vi "FPGA Main.vi"() -> ()   [LabVIEW 2018]
uses:
  <vilib>/Platform/TimedLoop/XDataNode/timing_clust.ctl
  <vilib>/Platform/TimedLoop/XDataNode/nitl_modes.ctl
  <vilib>/Platform/TimedLoop/XDataNode/wakeup.ctl
  <vilib>/rvi/Emulation/niFpgaGetClockAttributes.vi
  <vilib>/rvi/Emulation/niFpgaSctlEmulationGetInTimedLoop.vi
  <vilib>/rvi/Emulation/niFpgaEmulationReportErrorSimple.vi
  <vilib>/rvi/eio/common/nirviEmuTemplateMethod_errors.vi
  <vilib>/rvi/Emulation/niFpgaCriticalErrorInLSC.vi
  <vilib>/rvi/Emulation/niFpgaProcessEmulError.vi
  <vilib>/Platform/TimedLoop/XDataNode/XDataNode.xnode
  <vilib>/eio/EIONode/EIONode.xnode
  <vilib>/Platform/TimedLoop/XDataNode/XDNodeRunTimeDep.lvlib
panel:
  in  "Sample rate (Ticks) 1":i64=80
  in  "Sample rate (Ticks) 2":i64=80
  in  "Lower Threshold 2":i64
  in  "Anlalog input 2":refnum<k21>="ConnectorA/AI2"
  in  "Lower Threshold 1":i64
  in  "Anlalog input 1":refnum<k21>="ConnectorA/AI1"
  in  "chieu 2":bool=TRUE
  in  "chieu 1":bool=TRUE
  in  "start 2":bool
  in  "Fan Rotation 2":i64
  in  "Asix Rotation":i64
  in  "start 1":bool
  in  "reset count":bool
  out "coincedience":bool
  in  "reset":bool=TRUE
  in  "Gated-2  (ns)2":i64
  in  "Delay-1 (ns)":i64
  out "Count":i64
  out "signal out 2":bool
  out "signal out":bool
  in  "Delay-2 (ns)":i64
  in  "Gated-1  (ns)":i64
  in  "Digital input 2":refnum<k21>="ConnectorA/DIO1"
  in  "Digital input 1":refnum<k21>="ConnectorA/DIO0"
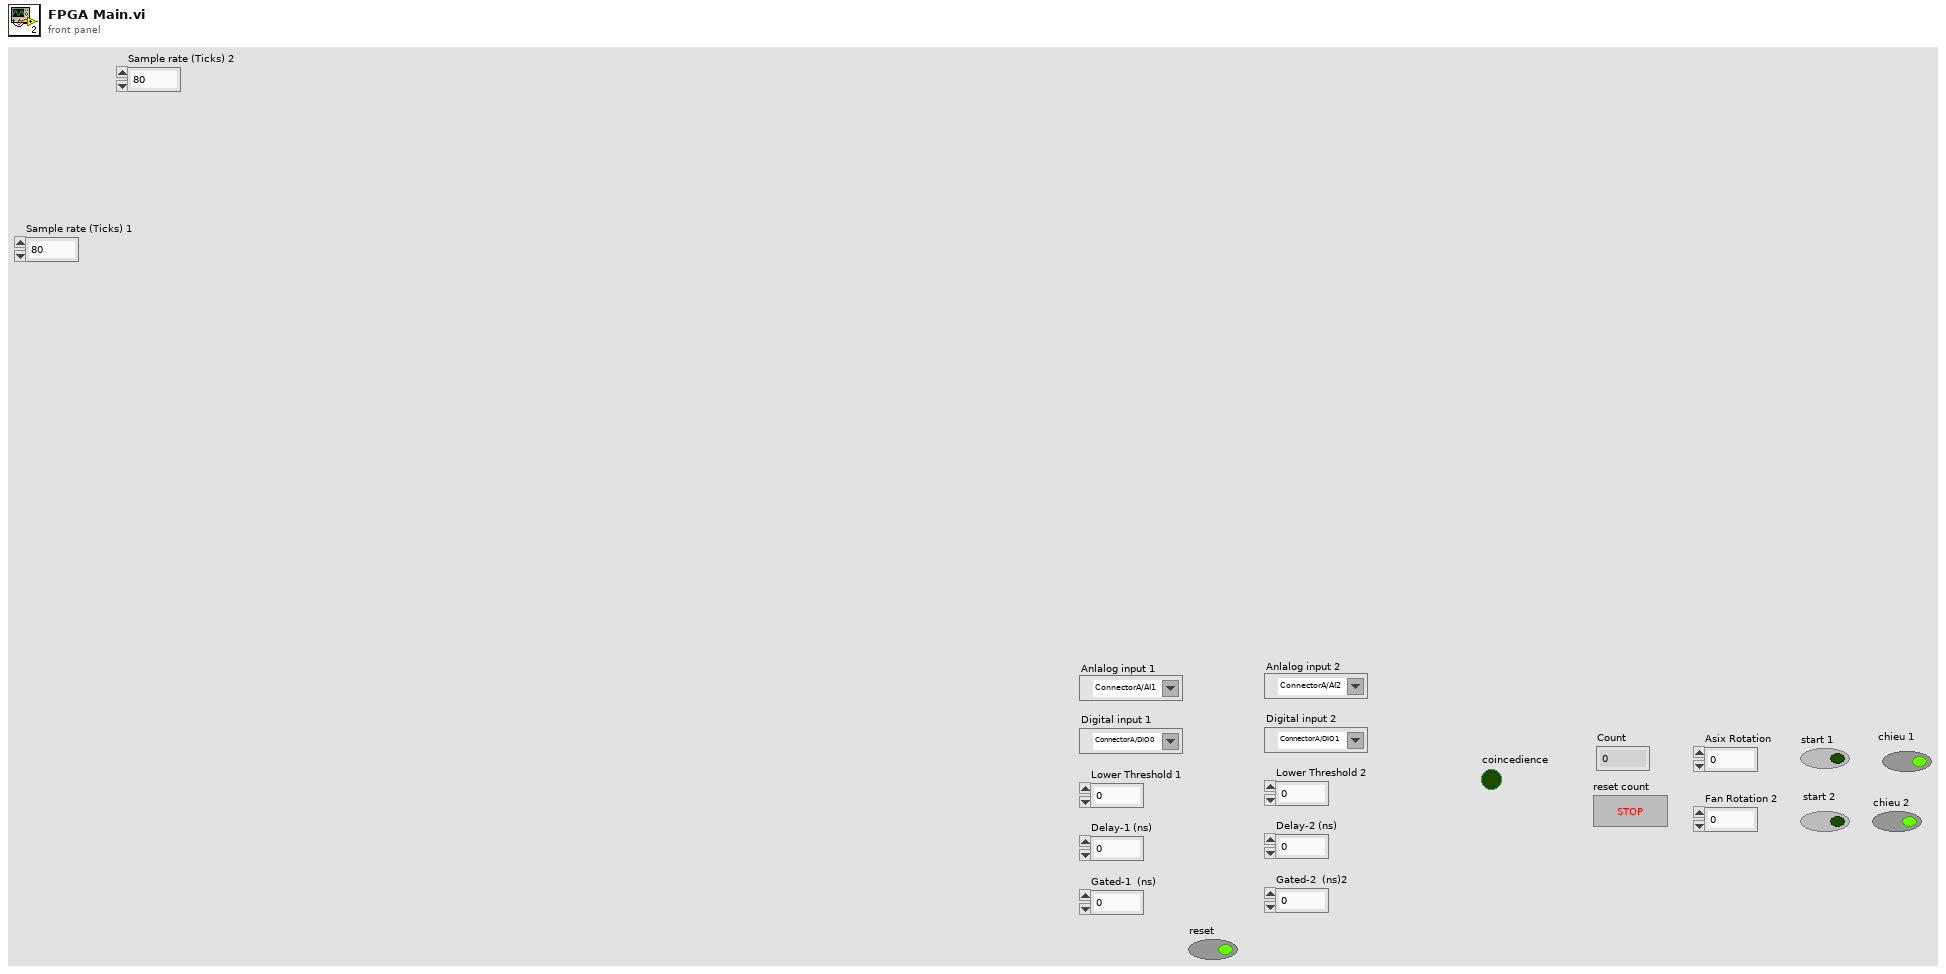
[diagram p1: front panel]
types:
  T1 = typedef "XDNodeRunTimeDep.lvlib/timing_clust.ctl" = cluster{"Expected End [f-1]":u64, "Actual End [f-1]":u64, "Finished Late? [f-1]":bool, "Expected End [i-1]":u64, "Actual End [i-1]":u64, "Finished Late? [i-1]":bool, "Expected Start [i]":u64, "Actual Start [i]":u64, "Expected Start [f]":u64, "Actual Start [f]":u64, "Source Name":string, "Structure Name":string, "Period":i64, "Deadline":i64, "Offset":i64, "Start":i64, "Priority":i32, "Timeout":i32, "Mode":T2, "Wakeup Reason":T3, "Error":errorcluster, "Source Type":string, "Secondary Source Type":string, "Global End Time":u64, "Global Start Time":u64, "Frame Duration":u64, "Iteration Duration":u64, "Assigned CPU":i32, "I/O Scan Engine Mode":u32}
  T2 = typedef "XDNodeRunTimeDep.lvlib/nitl_modes.ctl" = enum32{"No Change", "Process missed periods, maintain original phase", "Discard missed periods, maintain original phase", "Process missed periods, ignore original phase", "Discard missed periods, ignore original phase"}
  T3 = typedef "XDNodeRunTimeDep.lvlib/wakeup.ctl" = enum32{"Normal", "Aborted", "Asynchronous wakeup", "Timing source error", "Timed loop error", "Timeout"}
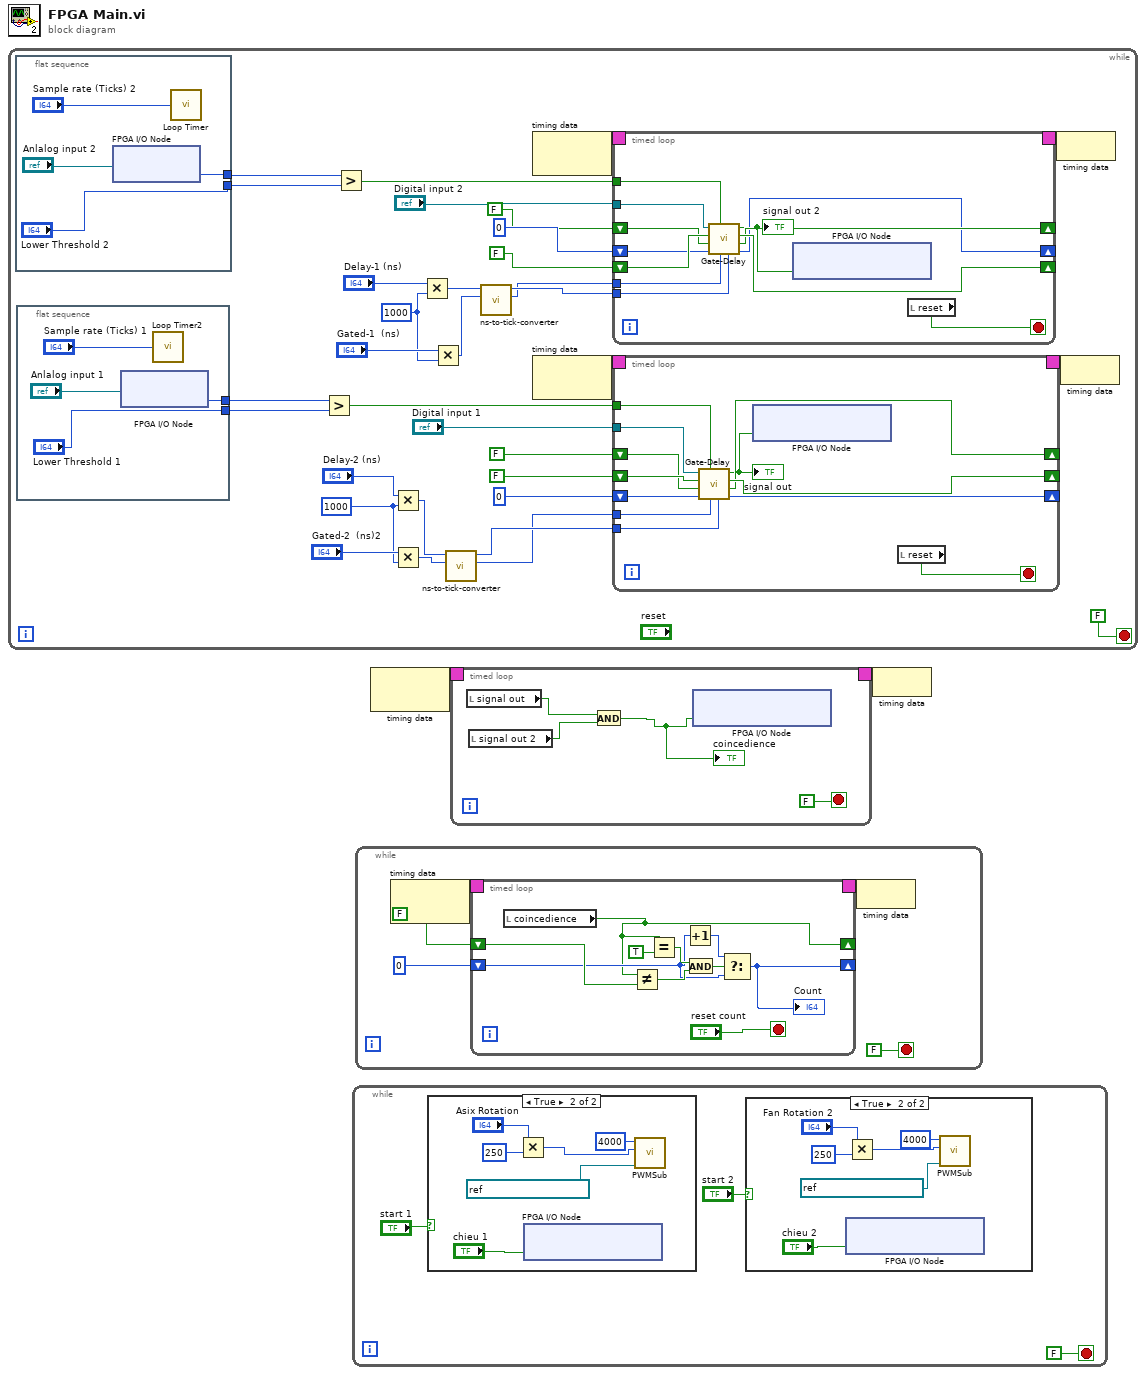
[diagram p0: block diagram]
diagram:
  n1 = while {
    stop <- FALSE stop-if-true
    w10 = i64 1000 ("y")
    w13 = i64 1000 ("y")
    n2 = flat-sequence {
      tunnel: [w40] -> w3
      tunnel: ["Lower Threshold 2"] -> w5
      frame #0 {
        n3 = xnode "FPGA I/O Node"("FPGA I/O In"="Anlalog input 2") -> ("I/O Item"=w40:u16)  [unwired: 1 out]
        n4 = call "Loop Timer"("Count(Ticks)"="Sample rate (Ticks) 2") -> ()  [unwired: 1 out]
      }
    }
    n5 = flat-sequence {
      tunnel: ["Lower Threshold 1"] -> w8
      tunnel: [w37] -> w7
      frame #0 {
        n6 = xnode "FPGA I/O Node"("FPGA I/O In"="Anlalog input 1") -> ("I/O Item"=w37:u16)  [unwired: 1 out]
        n7 = call "Loop Timer2"("Count(Ticks)"="Sample rate (Ticks) 1") -> ()  [unwired: 1 out]
      }
    }
    n8 = Greater?(x=w7, y=w8) -> (0:w6:bool)
    n9 = Greater?(x=w3, y=w5) -> (0:w4:bool)
    n10 = Multiply(x="Delay-2 (ns)", y=w10) -> (x*y=w11:i64)
    n11 = Multiply(x="Gated-2  (ns)2", y=w10) -> (x*y=w16:i64)
    n12 = Multiply(x="Delay-1 (ns)", y=w13) -> (x*y=w14:i64)
    n13 = Multiply(x="Gated-1  (ns)", y=w13) -> (x*y=w18:i64)
    n14 = call "ns-to-tick-converter.vi"("Gated-2  (ns)2"=w16, "Delay-2 (ns)"=w11) -> ("Numeric"=w22:i64, "Numeric 2"=w23:i64)  [unwired: 8 in]
    n15 = call "ns-to-tick-converter.vi"("Gated-2  (ns)2"=w18, "Delay-2 (ns)"=w14) -> ("Numeric"=w20:i64, "Numeric 2"=w21:i64)  [unwired: 8 in]
    n16 = node-c288() -> (w32:T1)  [unwired: 1 in]
    n17 = node-c288() -> (w35:T1)  [unwired: 1 in]
    n18 = timed-loop {
      timing: w32 -> [_]
      timing-out: [_] -> w31
      shift-right: [w53] -> _
      shift-left: FALSE ("adshift1'") -> [w54]
      tunnel: "Digital input 2" -> [w55]
      shift-right: [w51] -> _
      shift-left: FALSE ("adshift2'") -> [w52]
      shift-right: [w50] -> _
      shift-left: i64 0 ("adcounter'") -> [w49]
      tunnel: w20 -> [w48]
      tunnel: w21 -> [w45]
      tunnel: w4 -> [w44]
      stop <- w46 stop-if-true
      n19 = call "Gate-Delay.vi"("Delay (tick)"=w45, "Gated (tick)"=w48, "Analog input"=w44, "addcounter"=w49, "adshift2"=w52, "adshift1"=w54, "Refnum in"=w55) -> ("adcounter'"=w50:i64, "adshift2'"=w51:bool, "adshift1'"=w53:bool, "signal out"=w47:bool)  [unwired: 1 in]
      "signal out 2" <- w47
      n20 = xnode "FPGA I/O Node"("ConnectorA/DIO3"=w47) -> ()  [unwired: 1 in, 1 out]
      n21 = local read "reset"() -> (w46:bool)
    }
    n22 = timed-loop {
      timing: w35 -> [_]
      timing-out: [_] -> w34
      shift-right: [w69] -> _
      shift-left: FALSE ("adshift1'") -> [w70]
      tunnel: "Digital input 1" -> [w71]
      shift-right: [w67] -> _
      shift-left: FALSE ("adshift2'") -> [w68]
      shift-right: [w66] -> _
      shift-left: i64 0 ("adcounter'") -> [w65]
      tunnel: w23 -> [w64]
      tunnel: w22 -> [w62]
      tunnel: w6 -> [w60]
      stop <- w63 stop-if-true
      n23 = call "Gate-Delay.vi"("Delay (tick)"=w64, "Gated (tick)"=w62, "Analog input"=w60, "addcounter"=w65, "adshift2"=w68, "adshift1"=w70, "Refnum in"=w71) -> ("adcounter'"=w66:i64, "adshift2'"=w67:bool, "adshift1'"=w69:bool, "signal out"=w61:bool)  [unwired: 1 in]
      "signal out" <- w61
      n24 = xnode "FPGA I/O Node"("ConnectorA/DIO7"=w61) -> ()  [unwired: 1 in, 1 out]
      n25 = local read "reset"() -> (w63:bool)
    }
    n26 = node-c288(w31) -> ()
    n27 = node-c288(w34) -> ()
  }
  n28 = while {
    stop <- FALSE stop-if-true
    n29 = case shown="True" "start 1" {
      frame False {
      }
      frame True {
        n30 = Multiply(x="Asix Rotation", y=u32 250) -> (x*y=w88:u32)
        n31 = xnode "FPGA I/O Node"("ConnectorC/DIO2"="chieu 1") -> ()  [unwired: 1 in, 1 out]
        n32 = call "PWMSub.vi"("FPGA I/O In"=refnum<k21> "ConnectorC/DIO5", "Pluse"=w88, "Count(Ticks)"=u32 4000) -> ()  [unwired: 9 in]
      }
    }
    n33 = case shown="True" "start 2" {
      frame False {
      }
      frame True {
        n34 = xnode "FPGA I/O Node"("ConnectorC/DIO3"="chieu 2") -> ()  [unwired: 1 in, 1 out]
        n35 = Multiply(x="Fan Rotation 2", y=u32 250) -> (x*y=w81:u32)
        n36 = call "PWMSub.vi"("FPGA I/O In"=refnum<k21> "ConnectorC/DIO6", "Pluse"=w81, "Count(Ticks)"=u32 4000) -> ()  [unwired: 9 in]
      }
    }
  }
  n37 = while {
    stop <- FALSE stop-if-true
    n38 = node-c288() -> (w95:T1)  [unwired: 1 in]
    n39 = timed-loop {
      shift-right: [w99] -> _
      shift-left: i64 0 -> [w98]
      shift-right: [w96] -> _
      shift-left: FALSE ("x") -> [w100]
      timing: w95 -> [_]
      timing-out: [_] -> w94
      stop <- "reset count" stop-if-true
      n40 = local read "coincedience"() -> (w96:bool)
      n41 = Not Equal?(x=w96, y=w100) -> (x != y?=w104:bool)
      n42 = Equal?(x=w96, y=TRUE) -> (x = y?=w103:bool)
      n43 = Increment(x=w98) -> (x+1=w105:i64)
      n44 = And(x=w103, y=w104) -> (x .and. y?=w101:bool)
      n45 = Select(t=w105, s=w101, f=w98) -> (s? t:f=w99:i64)
      "Count" <- w99
    }
    n46 = node-c288(w94) -> ()
  }
  n47 = node-c288() -> (w2:T1)  [unwired: 1 in]
  n48 = timed-loop {
    timing: w2 -> [_]
    timing-out: [_] -> w1
    stop <- FALSE stop-if-true
    n49 = local read "signal out"() -> (w113:bool)
    n50 = local read "signal out 2"() -> (w112:bool)
    n51 = And(x=w113, y=w112) -> (x .and. y?=w110:bool)
    "coincedience" <- w110
    n52 = xnode "FPGA I/O Node"("ConnectorA/DIO2"=w110) -> ()  [unwired: 1 in, 1 out]
  }
  n53 = node-c288(w1) -> ()
